vi "MU Calibration Calculate Nonius Position.vi"(8 "error in (no error)":errorcluster, 9 "Continuous":bool, 10 "Calibration Unit":u32, 11 "analyzeResult":T1) -> (0 "error out":errorcluster, 2 "SingleturnPosition":dbl[](array[numeric]), 3 "Return Value":u64)   [LabVIEW 2017, in "MU_3SL_interface.lvlib"]
uses:
  MU_3SL_interface.lvlib
  handles/CalibrationAnalyzeResultHandle.ctl
  lib/MU_3SL_interface.dll
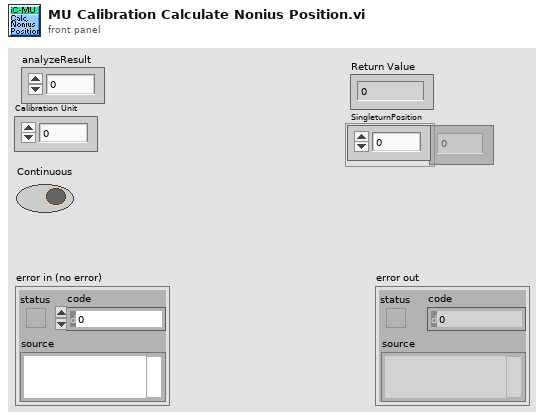
[diagram p1: front panel]
types:
  T1 = typedef "MU_3SL_interface.lvlib/CalibrationAnalyzeResultHandle.ctl" = u64
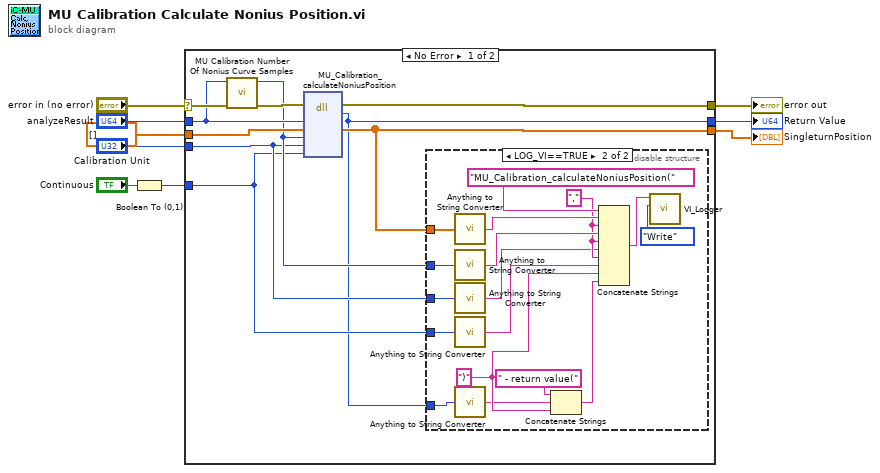
[diagram p0: block diagram]
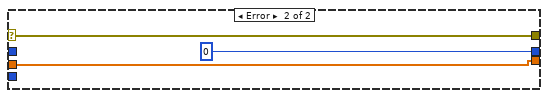
[diagram p3: hidden frame]
diagram:
  n1 = Boolean To (0,1)(Boolean="Continuous") -> (0, 1=w3:i16)
  n2 = case shown="No Error" "error in (no error)" {
    selector: "error in (no error)" -> [w18 w39]
    tunnel: "analyzeResult" -> [w17 _]
    tunnel: [w19 w39] -> w8
    tunnel: [w10 u64 0 ("return type")] -> w7
    tunnel: [w14 w37] -> w2
    tunnel: "Calibration Unit" -> [w12 _]
    tunnel: w3 -> [w11 _]
    tunnel: dbl[] [] ("SingleturnPosition") -> [w15 w37]
    frame No Error {
      n3 = call "MU Calibration Number Of Nonius Curve Samples.vi"("error in (no error)"=w18, "CalibrationAnalyzeResult"=w17) -> ("error out"=w16:errorcluster, "NumberOfNoniusCurveSamples"=w13:u64)  [unwired: 8 in]
      n4 = dll-call lib="C:/Users/bes/AppData/Roaming/work/mu_9so/icsubmodules/soft_mu_3sl_master/lv_interface/lib/MU_3SL_interface**.*" fn="MU_Calibration_calculateNoniusPosition"(error in=w16, "analyzeResult"=w17, "SingleturnPosition"=w15, "Singleturn Position Size"=w13, "Calibration Unit"=w12, "Continuous"=w11) -> (error out=w19:errorcluster, "Return Value"=w10:u64, "SingleturnPosition"=w14:dbl[])  [unwired: 6 in, 1 out]
      n5 = disable-structure shown="LOG_VI==TRUE" {
        disable-tunnel: w14 -> [_ w32]
        disable-tunnel: w13 -> [_ w30]
        disable-tunnel: w12 -> [_ w27]
        disable-tunnel: w11 -> [_ w26]
        disable-tunnel: w10 -> [_ w21]
        frame condition #0 {
        }
        frame condition #1 (active) {
          w28 = "," ("string")
          w23 = ")" ("string")
          n6 = call "Anything to String Converter.vi"("anything"=w32) -> ("String"=w31:string)
          n7 = call "Anything to String Converter.vi"("anything"=w30) -> ("String"=w29:string)
          n8 = call "Anything to String Converter.vi"("anything"=w27) -> ("String"=w25:string)
          n9 = call "Anything to String Converter.vi"("anything"=w26) -> ("String"=w24:string)
          n10 = call "Anything to String Converter.vi"("anything"=w21) -> ("String"=w20:string)
          n11 = Concatenate Strings(" - return value(" ("string"), w20, w23) -> (w22:string)
          n12 = Concatenate Strings("MU_Calibration_calculateNoniusPosition(" ("Info in"), w31, w28, w29, w28, w25, w28, w24, w23, w22) -> (w34:string)
          n13 = call "VI_Logger.vi"("Action (Read)"=enum16{"Write", "Read"}."Write", "Info in"=w34) -> ()  [unwired: 8 in, 2 out]
        }
      }
    }
    frame Error {
    }
  }
  "error out" <- w8
  "Return Value" <- w7
  "SingleturnPosition" <- w2
